vi "Initialization VI.vi"(8 "error in":errorcluster, 10 "Custom XML":string, 11 "Device Item Ref in":T1 format="%.0x") -> (0 "error out":errorcluster, 3 "Device Item Ref out":T1 format="%.0x")   [LabVIEW 2015, in "Scriptable Model Interface System Explorer.lvlib"]
uses:
  Scriptable Model Interface System Explorer.lvlib
  <vilib>/NI Veristand/Custom Device API/Custom Device Item Ref.ctl
  Shared/Constants.vi
  <vilib>/NI Veristand/Custom Device API/Custom Device API.lvlib
  Shared/Scriptable Model Interface Shared.lvlib
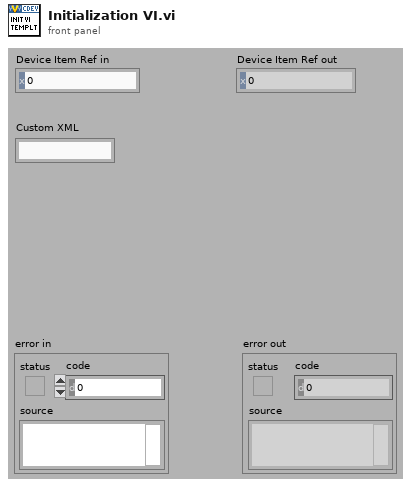
[diagram p1: front panel]
types:
  T1 = typedef "Custom Device API.lvlib/Custom Device Item Ref.ctl" = u64
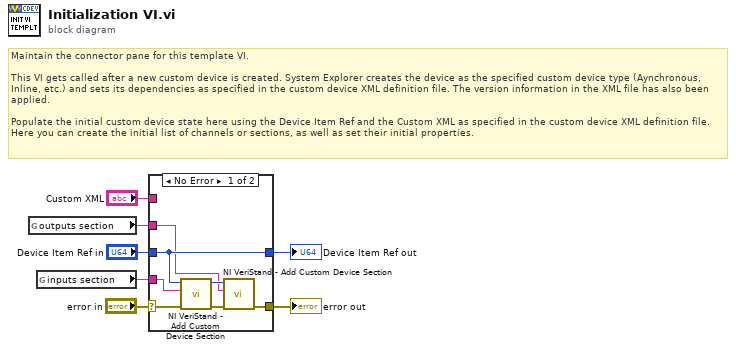
[diagram p0: block diagram]
diagram:
  # "Maintain the connector pane for this template VI.\n\nThis VI gets called after a new custom device is created. System Explorer creates the device as the specified custom device type (Aynchronous, Inline, etc.) and sets its dependencies as specified in the custom device XML definition file. The version information in the XML file has also been applied.\n\nPopulate the initial custom device state here using the Device Item Ref and the Custom XML as specified in the custom device XML definition file. Here you can create the initial list of channels or sections, as well as set their initial properties."
  n1 = global read "Constants.vi" "outputs section"() -> (w2:string)
  n2 = global read "Constants.vi" "inputs section"() -> (w1:string)
  n3 = case shown="No Error" "error in" {
    selector: "error in" -> [w11 w16]
    tunnel: [w10 w16] -> w7
    tunnel: [w14 w15] -> w5
    tunnel: "Device Item Ref in" -> [w14 w15]
    tunnel: "Custom XML" -> [_ _]
    tunnel: w2 -> [w9 _]
    tunnel: w1 -> [w8 _]
    frame No Error {
      n4 = call <vilib>:"NI VeriStand - Add Custom Device Section.vi"("error in (no error)"=w11, "Section Name"=w8, "Parent Ref in"=w14) -> ("error out"=w12:errorcluster, "Parent Ref out"=w13:T1)  [unwired: 5 in, 2 out]
      n5 = call <vilib>:"NI VeriStand - Add Custom Device Section.vi"("error in (no error)"=w12, "Section Name"=w9, "Parent Ref in"=w13) -> ("error out"=w10:errorcluster)  [unwired: 5 in, 3 out]
    }
    frame Error {
    }
  }
  "error out" <- w7
  "Device Item Ref out" <- w5
